vi "Handle setAllData.vi"(8 "error in (no error)":errorcluster, 10 "AllData":variant, 11 "Inst.TC in":refnum<class "Inst.TC.lvclass">) -> (0 "error out":errorcluster, 3 "Inst.TC out":refnum<class "Inst.TC.lvclass">)   [LabVIEW 2019, in "Inst.TC.lvclass"]
doc: "Override to handle incoming \"setAllData\" command for <b>your</b> Instrument"
uses:
  Inst.TC.lvclass
  Inst.TC.lvclass/Inst.TC.ctl
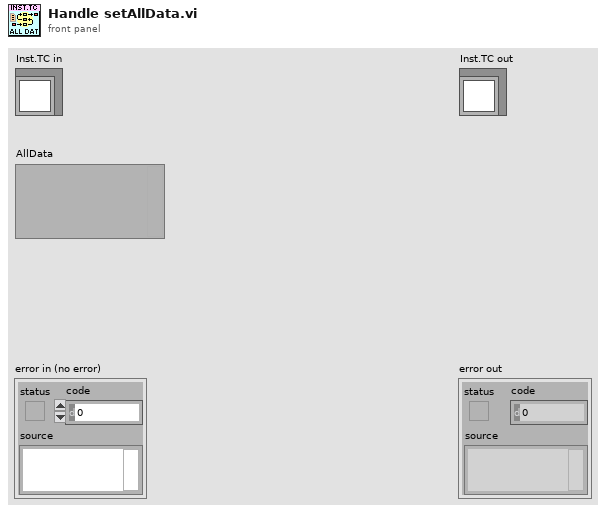
[diagram p1: front panel]
types:
  T1 = typedef "Inst.TC.lvclass/Inst.TC.getAll--Cluster.ctl" = cluster{"R":dbl[], "T":dbl[], "I":dbl[], "AVS Names":string, "Calibrations":string}
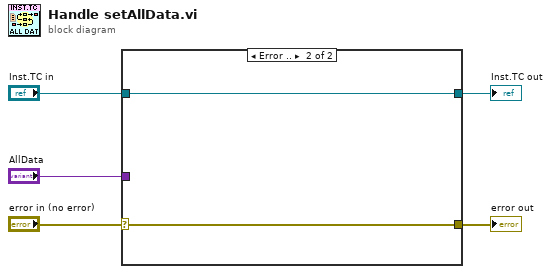
[diagram p0: block diagram]
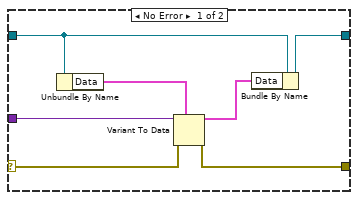
[diagram p2: hidden frame]
diagram:
  n1 = case shown="Error .." "error in (no error)" {
    selector: "error in (no error)" -> [w10 w14]
    tunnel: "AllData" -> [w11 _]
    tunnel: [w9 w14] -> w3
    tunnel: "Inst.TC in" -> [w8 w13]
    tunnel: [w6 w13] -> w1
    frame No Error {
      n2 = Unbundle By Name(w8) -> ("Data"=w12:T1)
      n3 = Variant To Data(error in=w10, type=w12, Variant=w11) -> (data=w7:T1, error out=w9:errorcluster)
      n4 = Bundle By Name(cluster=w8, "Data"=w7) -> (w6:refnum<class "Inst.TC.lvclass">)
    }
    frame Error {
    }
  }
  "error out" <- w3
  "Inst.TC out" <- w1
